vi "Hide Panel.vi"(8 "error in (no error)":errorcluster, 10 "Panel In":refnum<class "Panel.lvclass">, 11 "Manager in":refnum<class "Manager.lvclass">) -> (0 "error out":errorcluster, 2 "Panel":refnum<class "Panel.lvclass">, 3 "Manager out":refnum<class "Manager.lvclass">)   [LabVIEW 2014, in "OOPanel.lvlib" / "Manager.lvclass"]
uses:
  Manager.lvclass
  Panel/Panel.lvclass
  Panel/Visibility State.ctl
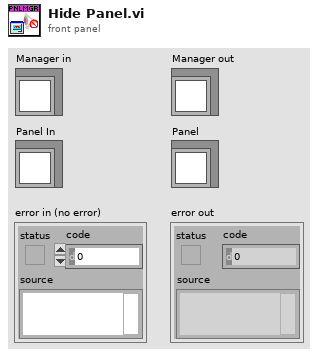
[diagram p1: front panel]
types:
  T1 = typedef "OOPanel.lvlib/Panel.lvclass/Visibility State.ctl" = enum16{"Idle", "Closed", "Hidden", "Visible", "Subpanel"}
  T2 = enum32{"Invalid", "Standard", "Closed", "Hidden", "Minimized", "Maximized"}
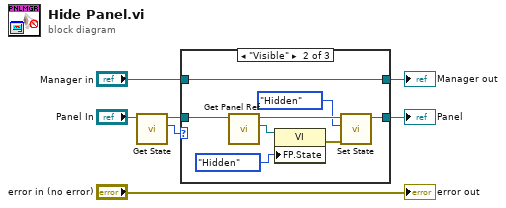
[diagram p0: block diagram]
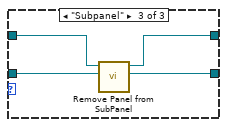
[diagram p3: hidden frame]
diagram:
  n1 = call "Get State.vi"("Panel in"="Panel In") -> ("State"=w4:T1, "Panel out"=w5:refnum<class "Panel.lvclass">)  [unwired: 8 in, 1 out]
  n2 = case shown="\"Visible\"" w4 {
    tunnel: w5 -> [w9 w16 w20]
    tunnel: "Manager in" -> [w8 w17 w21]
    tunnel: [w8 w17 w19] -> w2
    tunnel: [w9 w10 w18] -> w1
    frame Default {
      # "#ERROR?"
    }
    frame "Visible" {
      n3 = call "Get Panel Ref.vi"("Panel in"=w16) -> ("Panel Ref"=w15:refnum<vi>, "Panel out"=w13:refnum<class "Panel.lvclass">)  [unwired: 8 in, 1 out]
      n4 = property class="VI"(reference=w15, "FP.State"=T2."Hidden" ("Front Panel Window:State")) -> (error out=w12:errorcluster)  [unwired: 1 in, 1 out]
      n5 = call "Set State.vi"("error in (no error)"=w12, "State"=Visibility_State."Hidden", "Panel in"=w13) -> ("Panel out"=w10:refnum<class "Panel.lvclass">)  [unwired: 7 in, 1 out]
    }
    frame "Subpanel" {
      n6 = call "Remove Panel from SubPanel.vi"("Panel In"=w20, "Manager in"=w21) -> ("Panel"=w18:refnum<class "Panel.lvclass">, "Manager out"=w19:refnum<class "Manager.lvclass">)  [unwired: 7 in, 1 out]
    }
  }
  "Manager out" <- w2
  "Panel" <- w1
  "error out" <- "error in (no error)"
